vi "AILogger_FPGAtimeSync_tomerge.vi"() -> ()   [LabVIEW 2015]
uses:
  <vilib>/FPGAPlugInAG/cRIO-9114/niLvFpga_Open_cRIO-9114.vi
  <vilib>/rvi/interface/common/dynamic/niFpgaDynamicAddResources.vi
  <vilib>/Utility/error.llb/Error Cluster From Error Code.vi
  <vilib>/rvi/errors/niLvFpgaAdjustHostInterfaceError.vi
  <vilib>/FPGAPlugInAG/Dynamic/niLvFpga_Run_Dynamic.vi
  <vilib>/FPGAPlugInAG/Dynamic/niLvFpga_Close_Dynamic.vi
  <vilib>/rvi/interface/nirviOpenFPGA/nirviOpenFPGA.xnode
  FPGA Bitfiles/Canlogger3CHConv_FPGATarget_CANFrameFeedwith_OKF8Z1gjNso.lvbitx
  FPGA/CAN Frame Feed with Overflow Control (FPGA).vi
  <vilib>/rvi/interface/nirviReadWriteControl/nirviReadWriteControl.xnode
  <vilib>/rvi/interface/nirviMethod/nirviMethod.xnode
  <vilib>/rvi/interface/nirviCloseFPGA/nirviCloseFPGA.xnode
  <vilib>/rvi/errors/niLvFpgaMergeErrorWithErrorCode.vi
  examples copy/Timekeeper/FPGA Timekeeper.lvlib
  <vilib>/rvi/interface/Simulation/niFpgaSimulationCallBeginRW.vi
  <vilib>/FPGAPlugInAG/Dynamic/niLvFpga_ReadFifo_Dynamic.vi
  <vilib>/FPGAPlugInAG/Dynamic/niLvFpga_StartFifo_Dynamic.vi
  NiFpgaLv.dll
panel:
  out "Labview Time":timestamp[](array[timestamp])
  out "FPGA Timekeeper time (ns)":u64
  in  "millisecond multiple":u32=200
  out "time stamp error out":errorcluster
  in  "Time stamp stop":bool
  out "FPGA Timekeeper locked":bool
  out "offset from RT time (ns)":i32
  out "Elements Remaining":u32
  out "logged values":dbl[][](array[numeric])
  out "channel name(s) out":string[](array[string])
  in  "data layout (0:decimated)":enum16{"decimated", "interleaved"}(ring)
  out "RT loop time":u32
  out "AI 9205 loop rate":u32
  out "error out":errorcluster
  out "Timed Out?":bool
  in  "FPGA Loop rate (uSec)":u32=1000
  in  "stop":bool
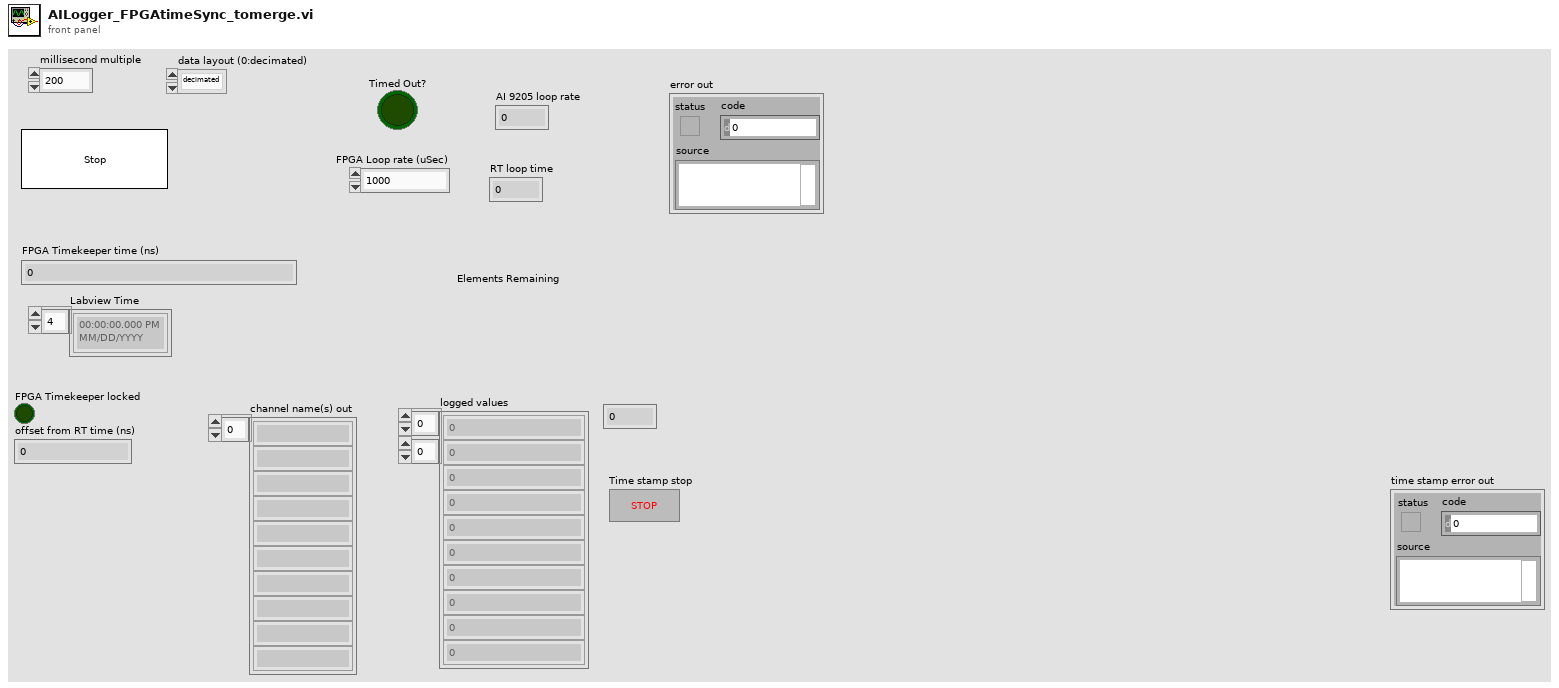
[diagram p1: front panel]
types:
  T1 = enum16{"open", "open or create", "create or replace", "create", "open (read-only)"}
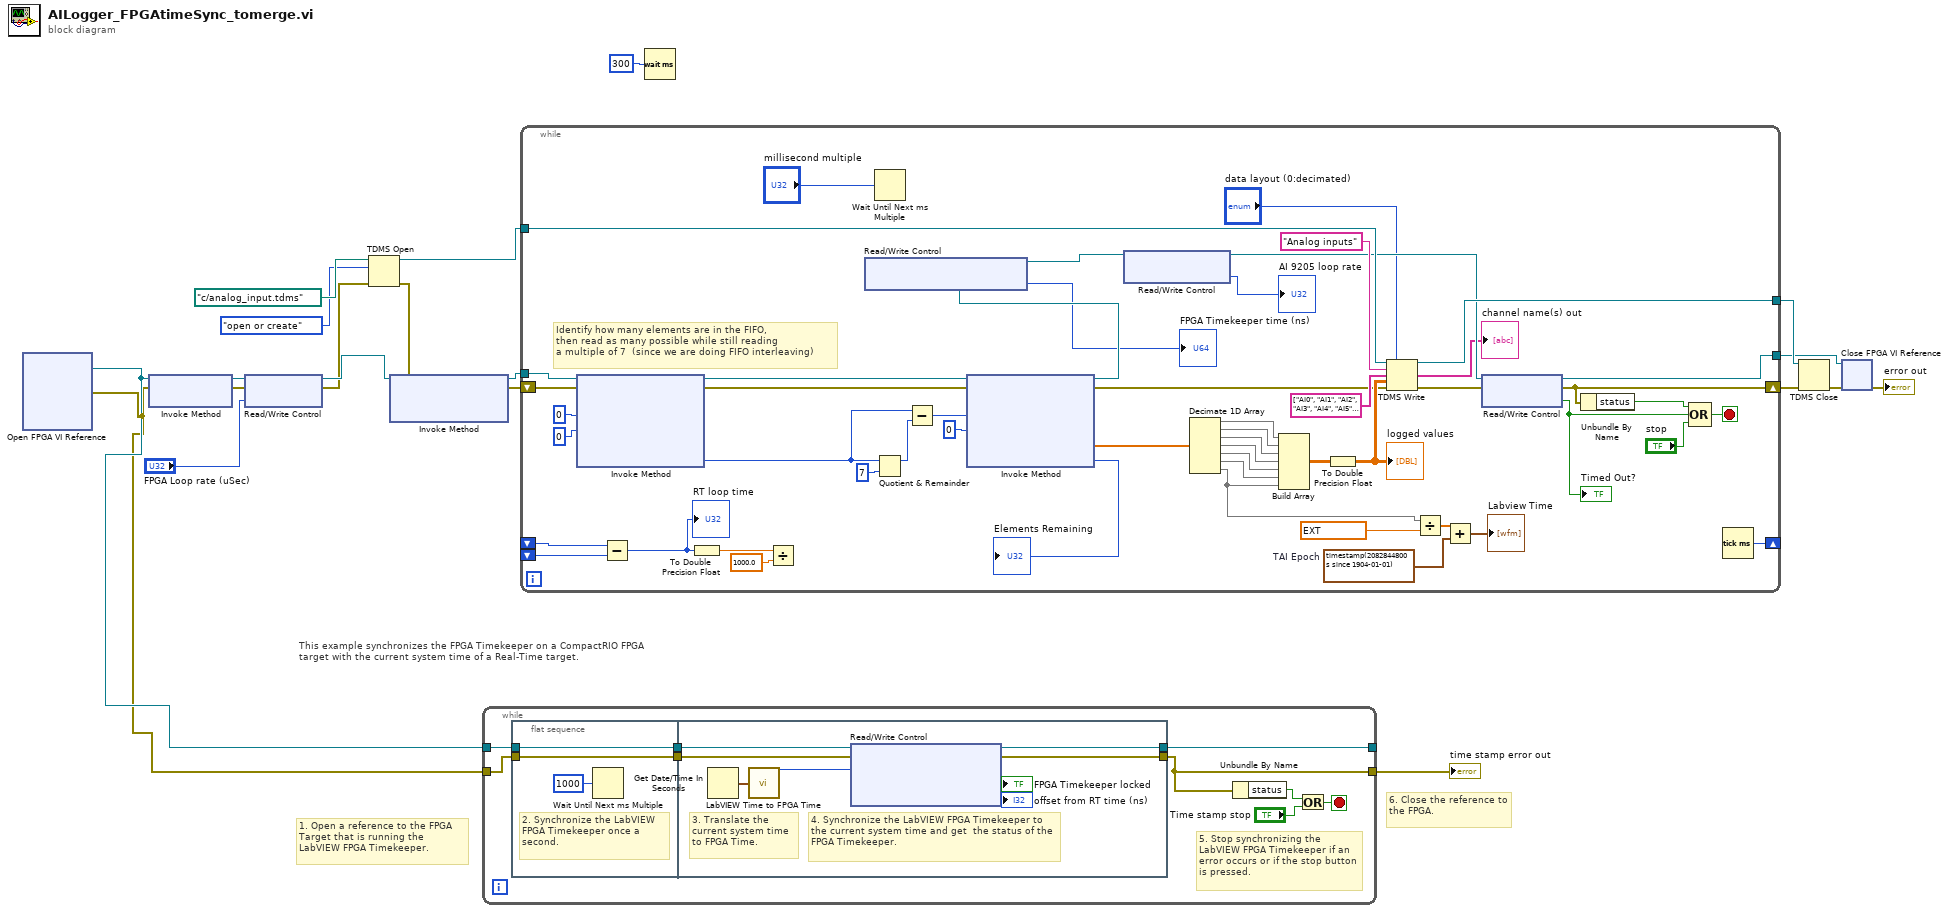
[diagram p0: block diagram]
diagram:
  # "This example synchronizes the FPGA Timekeeper on a CompactRIO FPGA target with the current system time of a Real-Time target."
  # "6. Close the reference to the FPGA."
  # "1. Open a reference to the FPGA\nTarget that is running the \nLabVIEW FPGA Timekeeper."
  n1 = xnode "Open FPGA VI Reference"() -> ("FPGA VI Reference Out"=w3:refnum<k20>, "error out"=w2:errorcluster)  [unwired: 2 in]
  n2 = xnode "Invoke Method"("FPGA VI Reference In"=w3, "error in"=w2) -> ("FPGA VI Reference Out"=w17:refnum<k20>, "error out"=w15:errorcluster)
  n3 = xnode "Read/Write Control"("FPGA VI Reference In"=w17, "error in"=w15, "Rate (uSec)"="FPGA Loop rate (uSec)") -> ("FPGA VI Reference Out"=w16:refnum<k20>, "error out"=w9:errorcluster)
  n4 = TDMS Open(8:w9, 10:T1."open or create" ("operation (0:open)"), 11:path "c:/analog_input.tdms" ("file path")) -> (0:w8:errorcluster, 3:w18:refnum<k34>)  [unwired: 4 in]
  n5 = xnode "Invoke Method"("FPGA VI Reference In"=w16, "error in"=w8) -> ("FPGA VI Reference Out"=w20:refnum<k20>, "error out"=w11:errorcluster)  [unwired: 1 in]
  n6 = while {
    tunnel: w3 -> [w29]
    tunnel: w2 -> [w24]
    tunnel: [w28] -> _
    tunnel: [w22] -> w4
    stop <- w26 stop-if-true
    # "5. Stop synchronizing the LabVIEW FPGA Timekeeper if an error occurs or if the stop button is pressed."
    n7 = flat-sequence {
      tunnel: w29 -> [w32]
      tunnel: [w32] -> w25
      tunnel: w24 -> [w31]
      tunnel: [w31] -> w23
      tunnel: [w40] -> w28
      tunnel: w25 -> [w37]
      tunnel: w23 -> [w36]
      tunnel: [w33] -> w22
      frame #0 {
        # "2. Synchronize the LabVIEW FPGA Timekeeper once a second."
        n8 = Wait Until Next ms Multiple(millisecond multiple=u32 1000) -> ()  [unwired: 1 out]
      }
      frame #1 {
        # "4. Synchronize the LabVIEW FPGA Timekeeper to the current system time and get  the status of the FPGA Timekeeper."
        # "3. Translate the current system time to FPGA Time."
        n9 = Get Date/Time In Seconds() -> (seconds since 1Jan1904=w35:timestamp)
        n10 = call "LabVIEW Time to FPGA Time.vi"("LabVIEW time"=w35) -> ("FPGA time (ns)"=w34:u64)
        n11 = xnode "Read/Write Control"("FPGA VI Reference In"=w37, "error in"=w36, "RT time (ns)"=w34) -> ("FPGA VI Reference Out"=w40:refnum<k20>, "error out"=w33:errorcluster, "FPGA Timekeeper locked"=→"FPGA Timekeeper locked":bool, "offset from RT time (ns)"=→"offset from RT time (ns)":i32)
      }
    }
    n12 = Unbundle By Name(w22) -> ("status"=w21:bool)
    n13 = Or(x=w21, y="Time stamp stop") -> (x .or. y?=w26:bool)
  }
  "time stamp error out" <- w4
  n14 = while {
    tunnel: w20 -> [w51]
    tunnel: [w88] -> w10
    tunnel: [w92] -> w19
    tunnel: w18 -> [w91]
    shift-right: [w84] -> w7
    shift-left: w11 -> [w57]
    shift-right: [w79] -> _
    shift-left: _ -> [w78]
    shift-left: _ -> [w77]
    stop <- w87 stop-if-true
    w45 = timestamp(2082844800 s since 1904-01-01)  # TAI Epoch
    # "Identify how many elements are in the FIFO, \nthen read as many possible while still reading\na multiple of 7  (since we are doing FIFO interleaving)"
    n15 = xnode "Invoke Method"("FPGA VI Reference In"=w51, "error in"=w57, "Number of Elements"=u32 0, "Timeout (ms)"=0) -> ("FPGA VI Reference Out"=w70:refnum<k20>, "error out"=w65:errorcluster, "Elements Remaining"=w68:u32)  [unwired: 1 out]
    n16 = Subtract(x=w78, y=w77) -> (x-y=w74:u32)
    "RT loop time" <- w74
    n17 = To Double Precision Float(number=w74) -> (double precision float=w73:dbl)
    n18 = Divide(x=w73, y=1000.0) -> ()  [unwired: 1 out]
    n19 = Wait Until Next ms Multiple(millisecond multiple="millisecond multiple") -> ()  [unwired: 1 out]
    n20 = Quotient & Remainder(x=w68, y=u32 7) -> (x-y*floor(x/y)=w69:u32)  [unwired: 1 out]
    n21 = Subtract(x=w68, y=w69) -> (x-y=w67:u32)
    n22 = xnode "Invoke Method"("FPGA VI Reference In"=w70, "error in"=w65, "Number of Elements"=w67, "Timeout (ms)"=0) -> ("FPGA VI Reference Out"=w48:refnum<k20>, "error out"=w52:errorcluster, "Data"=w60:sgl[], "Elements Remaining"=→"Elements Remaining":u32)
    n23 = xnode "Read/Write Control"("FPGA VI Reference In"=w48) -> ("FPGA VI Reference Out"=w47:refnum<k20>, "FPGA Timekeeper time (ns)"=→"FPGA Timekeeper time (ns)":u64)  [unwired: 1 in, 1 out]
    n24 = xnode "Read/Write Control"("FPGA VI Reference In"=w47) -> ("FPGA VI Reference Out"=w81:refnum<k20>, "AI 9205 loop rate"=→"AI 9205 loop rate":u32)  [unwired: 1 in, 1 out]
    n25 = Decimate 1D Array(w60) -> (w63:sgl[], w64:sgl[], w59:sgl[], w58:sgl[], w55:sgl[], w54:sgl[], w41:sgl[])
    n26 = Build Array(w63, w64, w59, w58, w55, w54, w41) -> (w62:sgl[][])
    n27 = To Double Precision Float(number=w62) -> (double precision float=w53:dbl[][])
    "logged values" <- w53
    n28 = TDMS Write(0:w91, 1:"data layout (0:decimated)", 5:"Analog inputs" ("group name in (Untitled)"), 7:string[] ["AI0", "AI1", "AI2", "AI3", "AI4", "AI5", "Time", "dt"] ("channel name(s) in (Untitled)"), 9:w53, 11:w52) -> (4:w92:refnum<k34>, 8:→"channel name(s) out":string[], 15:w83:errorcluster)  [unwired: 1 out]
    n29 = Divide(x=w41, y=ext 1000000000.0) -> (x/y=w44:ext[])
    n30 = Add(x=w44, y=w45) -> (x+y=→"Labview Time":timestamp[])
    n31 = xnode "Read/Write Control"("FPGA VI Reference In"=w81, "error in"=w83) -> ("FPGA VI Reference Out"=w88:refnum<k20>, "error out"=w84:errorcluster, "Timed Out?"=w82:bool)
    "Timed Out?" <- w82
    n32 = Unbundle By Name(w84) -> ("status"=w85:bool)
    n33 = Compound Arithmetic op=OR(w85, w82, "stop") -> (w87:bool)
    n34 = Tick Count (ms)() -> (millisecond timer value=w79:u32)
  }
  n35 = Wait (ms)(milliseconds to wait=u32 300) -> ()  [unwired: 1 out]
  n36 = TDMS Close(8:w7, 11:w19) -> (0:w6:errorcluster)  [unwired: 1 out]
  n37 = xnode "Close FPGA VI Reference"("FPGA VI Reference In"=w10, "error in"=w6) -> ("error out"=→"error out":errorcluster)
